vi "Gear Ratio (Steer).vi"(1 "Gear Ratio":dbl) -> (7 "Position Factor":dbl, 8 "Velocity Factor":dbl)   [LabVIEW 2025]
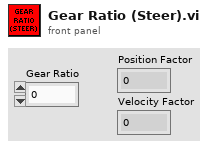
[diagram p1: front panel]
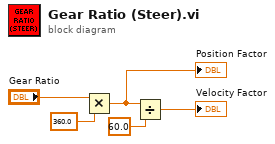
[diagram p0: block diagram]
diagram:
  n1 = Multiply(x="Gear Ratio", y=360.0) -> (x*y=w2:dbl)
  "Position Factor" <- w2
  n2 = Divide(x=w2, y=60.0) -> (x/y=→"Velocity Factor":dbl)
